vi "Image_capture_V1.0.vi"() -> ()   [LabVIEW 2024]
uses:
  <vilib>/userDefined/High Color/IMAQdx.ctl
  <vilib>/vision/driver/NI_Vision_Acquisition_Software.lvlib
panel:
  in  "File Path":path
  in  "Image Quality":u32=750 max=1000 step=10
  in  "Take image":bool
  out "error out 3":errorcluster
  out "error out 2":errorcluster
  out "Image":T1(plugin-control)
  out "error out":errorcluster
  in  "Camera selection":T2
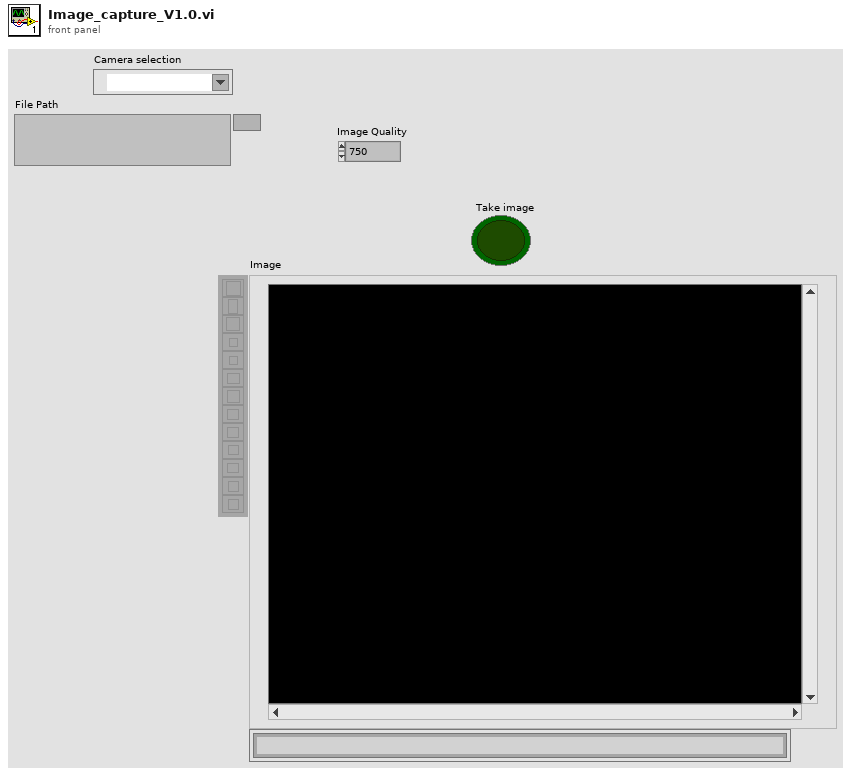
[diagram p1: front panel]
types:
  T1 = typedef "IMAQ Image.ctl" = refnum<image>
  T2 = typedef "IMAQdx.ctl" = refnum<k21>
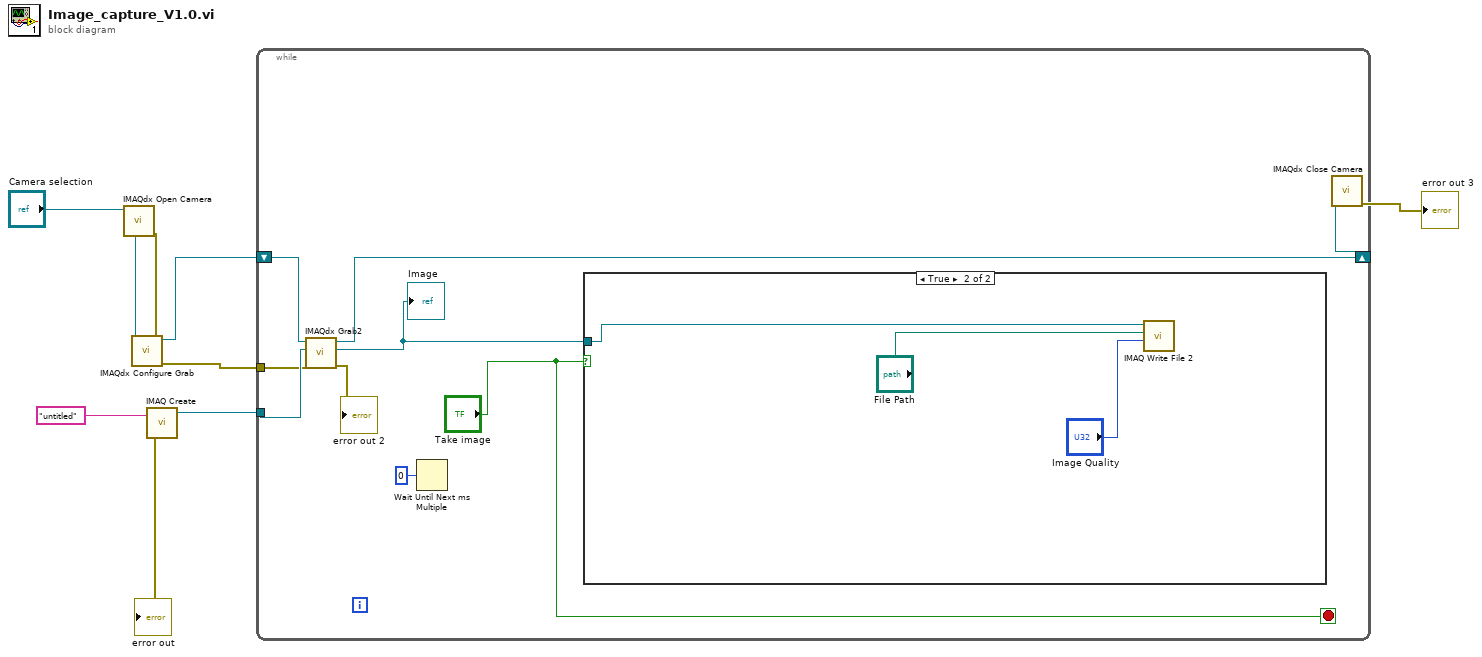
[diagram p0: block diagram]
diagram:
  n1 = call <vilib>:"IMAQdx Open Camera.vi"("Session In"="Camera selection") -> ("error out"=w8:errorcluster, "Session Out"=w10:T2)  [unwired: 9 in]
  n2 = call <vilib>:"IMAQdx Configure Grab.vi"("error in"=w8, "Session In"=w10) -> ("error out"=w2:errorcluster, "Session Out"=w7:T2)  [unwired: 8 in]
  n3 = call "IMAQ Create"("Image Name"="untitled") -> ("New Image"=w6:T1, "error out"=→"error out":errorcluster)  [unwired: 4 in]
  n4 = while {
    tunnel: w6 -> [w17]
    shift-right: [w16] -> w3
    shift-left: w7 -> [w18]
    tunnel: w2 -> [w15]
    stop <- "Take image" stop-if-true
    n5 = call <vilib>:"IMAQdx Grab2.vi"("error in"=w15, "Image In"=w17, "Session In"=w18) -> ("error out"=→"error out 2":errorcluster, "Image Out"=w12:T1, "Session Out"=w16:T2)  [unwired: 5 in, 1 out]
    "Image" <- w12
    n6 = Wait Until Next ms Multiple(millisecond multiple=u32 0) -> ()  [unwired: 1 out]
    n7 = case shown="True" "Take image" {
      tunnel: w12 -> [_ w21]
      frame False {
      }
      frame True {
        n8 = call-poly "IMAQ Write File 2"("Image Quality"="Image Quality", "File Path"="File Path", "Image"=w21) -> ()  [unwired: 7 in, 2 out]
      }
    }
  }
  n9 = call <vilib>:"IMAQdx Close Camera.vi"("Session In"=w3) -> ("error out"=→"error out 3":errorcluster)  [unwired: 10 in]
